vi "main.vi"() -> ()   [LabVIEW 2020]
doc: "该范例演示了通过VI查看其它VI的方法，还可运行和中止查看的VI。\n对于要中止的VI，应设置为可中止。对于无法中止的VI，可查看相关范例。"
uses:
  global/GlobalVariable.vi
  global/SettingVariable.vi
  <vilib>/Utility/config.llb/Write Key (Path).vi
  utilities/NI_modbus.llb/MB Ethernet Master Query Write Multiple Registers (poly).vi
  utilities/NI_modbus.llb/MB Ethernet Master Query Read Input Registers (poly).vi
  <vilib>/Utility/config.llb/NI_LVConfig.lvlib
panel:
  in  "退出":bool
  in  "Measure Square":bool
  in  "Physics Parameters Square":bool
  in  "Open Square":bool
  in  "Home Square":bool
  out "时间":string
  out "日期":string
  in  "MainPanel":enum32{"logo"}(tab)
  out "P2_8":dbl
  out "P2_7":dbl
  out "P2_6":dbl
  out "P2_5":dbl
  out "P2_4":dbl
  out "P2_3":dbl
  out "P2_2":dbl
  out "P2_1":dbl
  out "电流 2":dbl(slide)=1.0 scale=1e-13..0.0001 scale format="%#_2e"
  out "电流 1":dbl(slide)=1.0 scale=1e-13..0.0001 scale format="%#_2e"
  out "电压8":dbl(knob) caption="Gauge" scale=1.0..5.0
  out "电压7":dbl(knob)=1.0 caption="Gauge" scale=1.0..5.0
  out "电压6":dbl(knob)=1.0 caption="Gauge" scale=1.0..5.0
  out "电压5":dbl(knob)=1.0 caption="Gauge" scale=1.0..5.0
  out "电压4":dbl(knob)=1.0 caption="Gauge" scale=1.0..5.0
  out "电压3":dbl(knob)=1.0 caption="Gauge" scale=1.0..5.0
  out "电压2":dbl(knob) caption="Gauge" scale=1.0..5.0
  out "电压1":dbl(knob) caption="Gauge" scale=1.0..5.0
  in  "网络链接":bool
  # "iRho-100型反应性仪"
  # "Network"
  # "Current1"
  # "Current2"
  # "Voltage Output"
  # "Voltage Input"
  # "AC220V/50Hz"
  # "Ground"
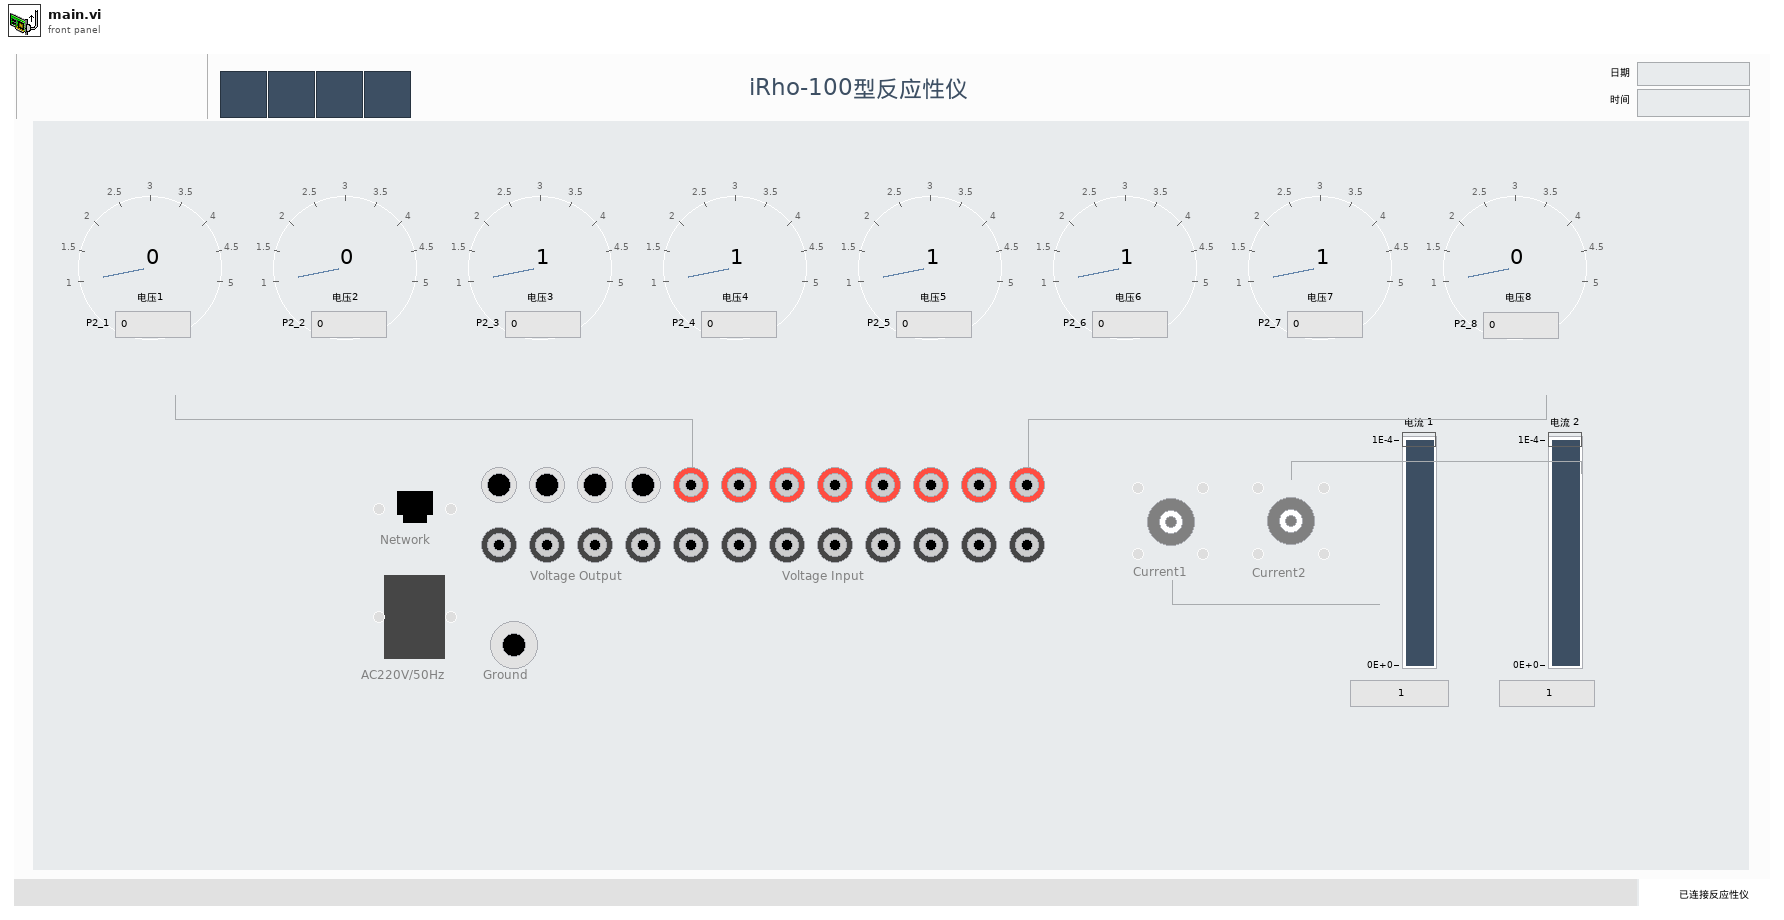
[diagram p1: front panel]
types:
  T1 = enum8{"Enabled", "Disabled", "Disabled and Grayed Out"}
  T2 = enum32{"Invalid", "Standard", "Closed", "Hidden", "Minimized", "Maximized"}
  T3 = cluster{"switch":bool, "name":string, "voltage upper":i32, "voltage lower":i32, "physics upper":dbl, "physics lower":dbl, "scale":u16}[]
  T4 = typedef "NI_LVConfig.lvlib/Config Data RefNum.ctl" = refnum<k1>
  T5 = enum32{"invalid app kind", "Development System", "Run Time System", "Student Edition", "Embedded LabVIEW", "Evaluation", "Custom"}
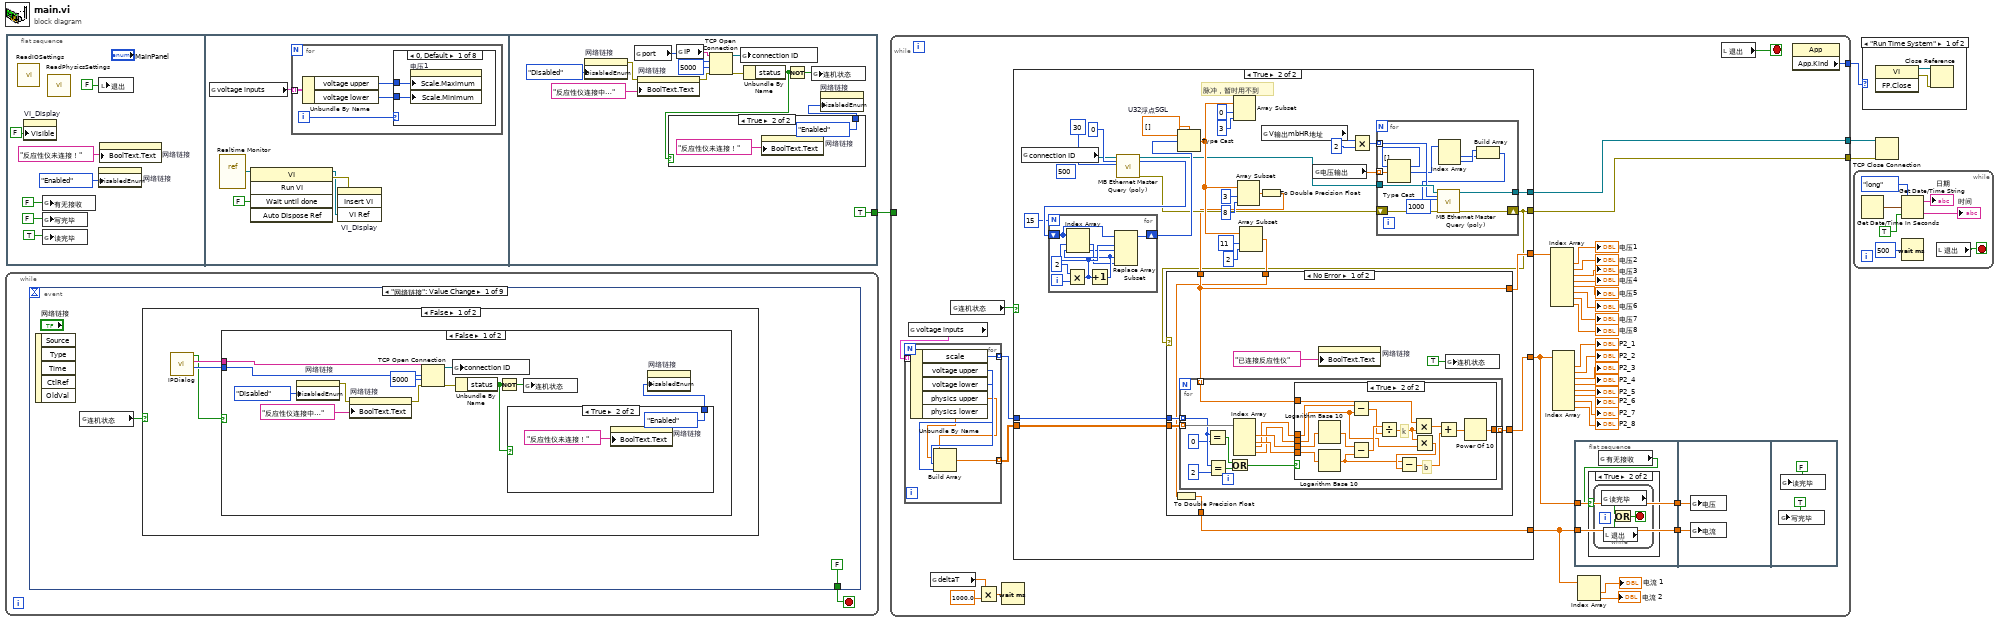
[diagram p0: block diagram]
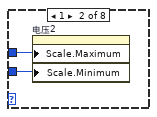
[diagram p2: hidden frame]
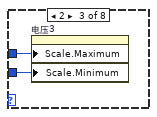
[diagram p3: hidden frame]
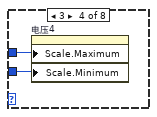
[diagram p4: hidden frame]
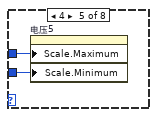
[diagram p5: hidden frame]
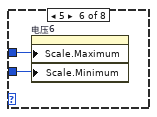
[diagram p6: hidden frame]
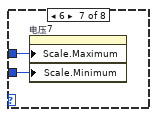
[diagram p7: hidden frame]
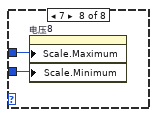
[diagram p8: hidden frame]
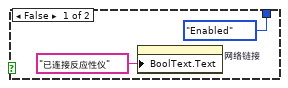
[diagram p9: hidden frame]
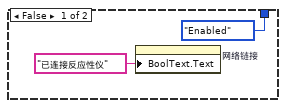
[diagram p10: hidden frame]
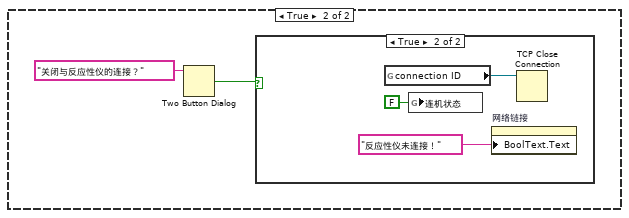
[diagram p12: hidden frame]
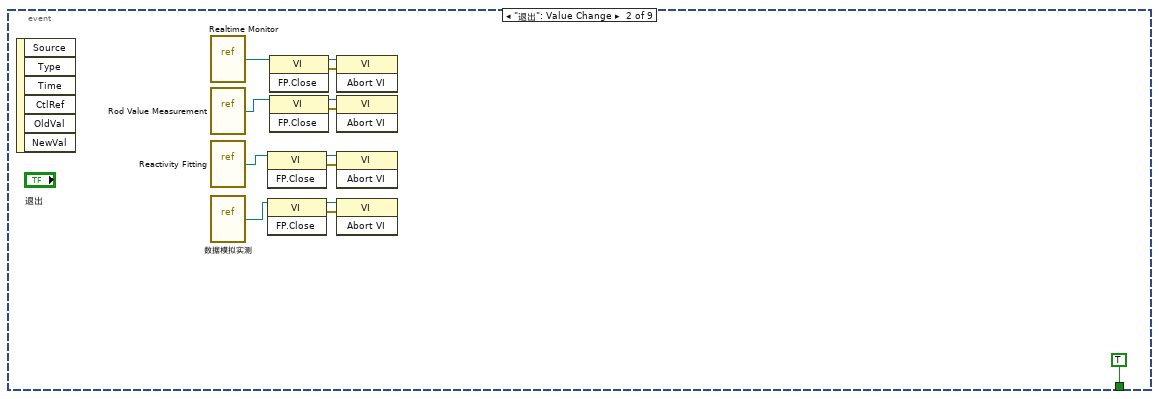
[diagram p14: hidden frame]
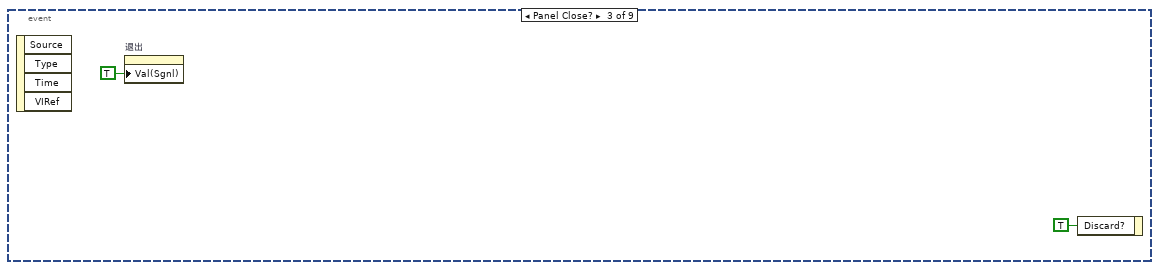
[diagram p15: hidden frame]
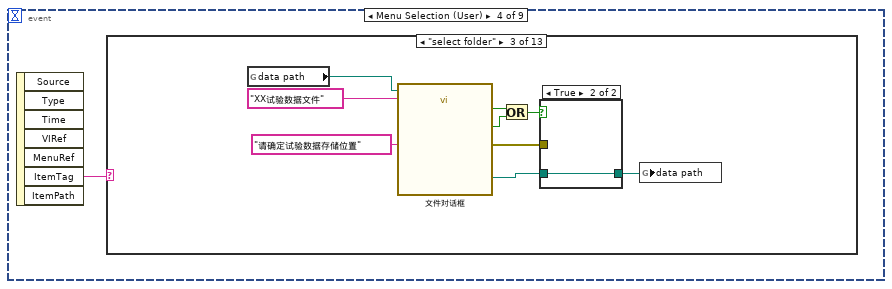
[diagram p16: hidden frame]
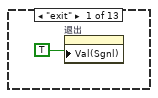
[diagram p17: hidden frame]
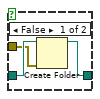
[diagram p19: hidden frame]
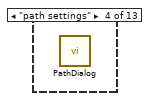
[diagram p20: hidden frame]
diagram:
  n1 = while {
    stop <- w5 stop-if-true
    n2 = event shown="[0] \"网络链接\": Value Change" {
      selector: _ -> [_ _ _ _ _ _ _ _ _]
      dyn-events: _ -> [_ _ _ _ _ _ _ _ _]
      timeout: _ -> [_ _ _ _ _ _ _ _ _]
      tunnel: [FALSE TRUE _ _ _ _ _ _ _] -> w5
      event "网络链接": Value Change {
        n3 = event-data() -> ()  [unwired: 1 in, 5 out]
        n4 = global read "GlobalVariable.vi" "连机状态"() -> (w6:bool)
        n5 = case shown="False" w6 {
          frame False {
            n6 = call "IPDialog.vi"() -> ("port"=w10:u16, "IP"=w9:string, "Cancelled?"=w8:bool)  [unwired: 9 in]
            n7 = case shown="False" w8 {
              tunnel: w10 -> [w14 _]
              tunnel: w9 -> [w13 _]
              frame False {
                n8 = property on="网络链接" class="Bool"("DisabledEnum"=T1."Disabled" ("Disabled")) -> (error out=w17:errorcluster)  [unwired: 2 in, 1 out]
                n9 = property on="网络链接" class="Bool"(error in=w17, "BoolText.Text"="反应性仪连接中…" ("Boolean Text.Text")) -> (error out=w19:errorcluster)  [unwired: 1 in, 1 out]
                n10 = TCP Open Connection(address=w13, remote port or service name=w14, timeout ms (60000)=5000, error in (no error)=w19) -> (connection ID=w18:refnum<k5>, error out=w15:errorcluster)  [unwired: 1 out]
                n11 = global write "GlobalVariable.vi" "connection ID"(w18) -> ()
                n12 = Unbundle By Name(w15) -> ("status"=w20:bool)
                n13 = Not(x=w20) -> (.not. x?=w21:bool)
                n14 = case shown="True" w20 {
                  tunnel: [T1."Enabled" ("Disabled") T1."Enabled" ("Disabled")] -> w12
                  frame False {
                    n15 = property on="网络链接" class="Bool"("BoolText.Text"="已连接反应性仪") -> ()  [unwired: 2 in, 2 out]
                  }
                  frame True {
                    n16 = property on="网络链接" class="Bool"("BoolText.Text"="反应性仪未连接！") -> ()  [unwired: 2 in, 2 out]
                  }
                }
                n17 = global write "GlobalVariable.vi" "连机状态"(w21) -> ()
                n18 = property on="网络链接" class="Bool"("DisabledEnum"=w12) -> ()  [unwired: 2 in, 2 out]
              }
              frame True {
              }
            }
          }
          frame True {
            n19 = Two Button Dialog(message="关闭与反应性仪的连接？") -> (T button?=w27:bool)  [unwired: 2 in]
            n20 = case shown="True" w27 {
              frame False {
              }
              frame True {
                n21 = global read "GlobalVariable.vi" "connection ID"() -> (w31:refnum<k5>)
                n22 = global write "GlobalVariable.vi" "连机状态"(FALSE ("连机状态")) -> ()
                n23 = property on="网络链接" class="Bool"("BoolText.Text"="反应性仪未连接！" ("Boolean Text.Text")) -> ()  [unwired: 2 in, 2 out]
                n24 = TCP Close Connection ("关闭TCP连接")(connection ID=w31) -> ()  [unwired: 1 in, 3 out]
              }
            }
          }
        }
      }
      event "退出": Value Change {
        n25 = event-data() -> ()  [unwired: 1 in, 6 out]
        n26 = vi-ref "Realtime Monitor.vi"() -> (w43:refnum<vi>)
        n27 = vi-ref "Rod Value Measurement.vi"() -> (w42:refnum<vi>)
        n28 = vi-ref "Reactivity Fitting.vi"() -> (w40:refnum<vi>)
        n29 = vi-ref "数据模拟实测.vi"() -> (w41:refnum<vi>)
        n30 = invoke class="VI" method="FP.Close"(reference=w40) -> (reference out=w35:refnum<vi>, error out=w34:errorcluster)  [unwired: 2 in, 1 out]
        n31 = invoke class="VI" method="FP.Close"(reference=w41) -> (reference out=w33:refnum<vi>, error out=w32:errorcluster)  [unwired: 2 in, 1 out]
        n32 = invoke class="VI" method="FP.Close"(reference=w43) -> (reference out=w39:refnum<vi>, error out=w38:errorcluster)  [unwired: 2 in, 1 out]
        n33 = invoke class="VI" method="FP.Close"(reference=w42) -> (reference out=w37:refnum<vi>, error out=w36:errorcluster)  [unwired: 2 in, 1 out]
        n34 = invoke class="VI" method="Abort VI"(reference=w39, error in=w38) -> ()  [unwired: 1 in, 3 out]
        n35 = invoke class="VI" method="Abort VI"(reference=w37, error in=w36) -> ()  [unwired: 1 in, 3 out]
        n36 = invoke class="VI" method="Abort VI"(reference=w35, error in=w34) -> ()  [unwired: 1 in, 3 out]
        n37 = invoke class="VI" method="Abort VI"(reference=w33, error in=w32) -> ()  [unwired: 1 in, 3 out]
      }
      event Panel Close? {
        n38 = event-data() -> ()  [unwired: 1 in, 4 out]
        n39 = property on="退出" class="Bool (strict)"("Val(Sgnl)"=TRUE ("Value (Signaling)")) -> ()  [unwired: 2 in, 2 out]
        n40 = event-data("Discard?"=TRUE) -> ()  [unwired: 1 in, 1 out]
      }
      event Menu Selection (User) {
        n41 = event-data() -> ("ItemTag"=w47:string)  [unwired: 1 in, 6 out]
        n42 = case shown="\"select folder\"" w47 {
          frame "exit" {
            n43 = property on="退出" class="Bool (strict)"("Val(Sgnl)"=TRUE) -> ()  [unwired: 2 in, 2 out]
          }
          frame Default {
          }
          frame "select folder" {
            n44 = global read "SettingVariable.vi" "data path"() -> (w50:path)
            n45 = call "文件对话框"("start path"=w50, "prompt"="请确定试验数据存储位置", "default name"="XX试验数据文件") -> ("selected path"=w57:path, "exists"=w55:bool, "cancelled"=w53:bool, "error out"=w56:errorcluster)  [unwired: 9 in]
            n46 = Or(x=w55, y=w53) -> (x .or. y?=w54:bool)
            n47 = case shown="True" w54 {
              tunnel: w57 -> [w60 w61]
              tunnel: w56 -> [w59 _]
              tunnel: [w58 w61] -> w49
              frame False {
                n48 = Create Folder(path (use dialog)=w60, error in=w59) -> (created path=w58:path)  [unwired: 1 in, 2 out]
              }
              frame True {
              }
            }
            n49 = global write "SettingVariable.vi" "data path"(w49) -> ()
          }
          frame "path settings" {
            n50 = call "PathDialog.vi"() -> ()  [unwired: 11 in, 1 out]
          }
          frame "physics settings" {
            n51 = call "PhysicsDialog.vi"() -> ()  [unwired: 1 in]
          }
          frame "input settings" {
            n52 = call "InputDialog.vi"() -> ("Cancelled?"=w62:bool)  [unwired: 9 in]
            n53 = case shown="True" w62 {
              frame False {
              }
              frame True {
                n54 = global read "SettingVariable.vi" "voltage inputs"() -> (w63:T3)
                n55 = for {
                  tunnel: w63 -> [w67] mode=indexing
                  i -> [w66]
                  n56 = Unbundle By Name(w67) -> ("voltage upper"=w65:i32, "voltage lower"=w64:i32)
                  n57 = case shown="0, Default" w66 {
                    tunnel: w65 -> [w69 w71 w73 w75 w77 w79 w81 w83]
                    tunnel: w64 -> [w68 w70 w72 w74 w76 w78 w80 w82]
                    frame 0, Default {
                      n58 = property on="电压1" class="Knob (strict)"("Scale.Maximum"=w69, "Scale.Minimum"=w68) -> ()  [unwired: 2 in, 2 out]
                    }
                    frame 1 {
                      n59 = property on="电压2" class="Knob (strict)"("Scale.Maximum"=w71, "Scale.Minimum"=w70) -> ()  [unwired: 2 in, 2 out]
                    }
                    frame 2 {
                      n60 = property on="电压3" class="Knob (strict)"("Scale.Maximum"=w73, "Scale.Minimum"=w72) -> ()  [unwired: 2 in, 2 out]
                    }
                    frame 3 {
                      n61 = property on="电压4" class="Knob (strict)"("Scale.Maximum"=w75, "Scale.Minimum"=w74) -> ()  [unwired: 2 in, 2 out]
                    }
                    frame 4 {
                      n62 = property on="电压5" class="Knob (strict)"("Scale.Maximum"=w77, "Scale.Minimum"=w76) -> ()  [unwired: 2 in, 2 out]
                    }
                    frame 5 {
                      n63 = property on="电压6" class="Knob (strict)"("Scale.Maximum"=w79, "Scale.Minimum"=w78) -> ()  [unwired: 2 in, 2 out]
                    }
                    frame 6 {
                      n64 = property on="电压7" class="Knob (strict)"("Scale.Maximum"=w81, "Scale.Minimum"=w80) -> ()  [unwired: 2 in, 2 out]
                    }
                    frame 7 {
                      n65 = property on="电压8" class="Knob (strict)"("Scale.Maximum"=w83, "Scale.Minimum"=w82) -> ()  [unwired: 2 in, 2 out]
                    }
                  }
                }
              }
            }
          }
          frame "output settings" {
            n66 = call "OutputDialog.vi"() -> ()  [unwired: 11 in, 1 out]
          }
          frame "homepage" {
            n67 = property on="VI_Display" class="SubPnl"("Visible"=FALSE) -> ()  [unwired: 2 in, 2 out]
          }
          frame "monitor" {
            n68 = property on="VI_Display" class="SubPnl"("Visible"=TRUE) -> ()  [unwired: 2 in, 2 out]
          }
          frame "rod measurement" {
            n69 = vi-ref "Rod Value Measurement.vi"() -> (w88:refnum<vi>)
            n70 = invoke class="VI" method="FP.Open"(reference=w88, "Activate"=TRUE ("Activate?"), "State"=T2."Standard") -> (reference out=w89:refnum<vi>)  [unwired: 2 in, 4 out]
            n71 = invoke class="VI" method="Run VI"(reference=w89, "Wait until done"=FALSE ("Wait Until Done"), "Auto Dispose Ref"=FALSE ("Auto Dispose Reference")) -> ()  [unwired: 2 in, 5 out]
          }
          frame "reactivity fitting" {
            n72 = vi-ref "Reactivity Fitting.vi"() -> (w94:refnum<vi>)
            n73 = invoke class="VI" method="FP.Open"(reference=w94, "Activate"=TRUE ("Activate?"), "State"=T2."Standard") -> (reference out=w95:refnum<vi>)  [unwired: 2 in, 4 out]
            n74 = invoke class="VI" method="Run VI"(reference=w95, "Wait until done"=FALSE ("Wait Until Done"), "Auto Dispose Ref"=FALSE ("Auto Dispose Reference")) -> ()  [unwired: 2 in, 5 out]
          }
          frame "history simulation" {
            n75 = vi-ref "数据模拟实测.vi"() -> (w100:refnum<vi>)
            n76 = invoke class="VI" method="FP.Open"(reference=w100, "Activate"=TRUE ("Activate?"), "State"=T2."Standard") -> (reference out=w101:refnum<vi>)  [unwired: 2 in, 4 out]
            n77 = invoke class="VI" method="Run VI"(reference=w101, "Wait until done"=FALSE ("Wait Until Done"), "Auto Dispose Ref"=FALSE ("Auto Dispose Reference")) -> ()  [unwired: 2 in, 5 out]
          }
          frame "about" {
            n78 = call "About.vi"() -> ()  [unwired: 1 in]
          }
        }
      }
      event "Home Square": Value Change {
        n79 = event-data() -> ()  [unwired: 1 in, 6 out]
        n80 = property on="VI_Display" class="SubPnl"("Visible"=FALSE) -> ()  [unwired: 2 in, 2 out]
      }
      event "Measure Square": Value Change {
        n81 = event-data() -> ()  [unwired: 1 in, 6 out]
        n82 = property on="VI_Display" class="SubPnl"("Visible"=TRUE) -> ()  [unwired: 2 in, 2 out]
      }
      event "Open Square": Value Change {
        n83 = event-data() -> ()  [unwired: 1 in, 6 out]
        n84 = global read "SettingVariable.vi" "data path"() -> (w106:path)
        n85 = call <vilib>:"Space Constant.vi"() -> ("String"=w120:string)
        n86 = Path To String(path=w106) -> (string=w117:string)
        n87 = Concatenate Strings("explorer" ("字符串"), w120, w117) -> (w118:string)
        n88 = call <vilib>:"System Exec.vi"("command line"=w118) -> ()  [unwired: 7 in, 4 out]
        n89 = call <vilib>:"Application Directory.vi"() -> ("Application Directory"=w112:path)
        n90 = Build Path(base path=w112, name or relative path=path "configure.ini") -> (appended path=w113:path)
        n91 = call <vilib>:"Open Config Data.vi"("configuration file path"=w113) -> ("error out"=w115:errorcluster, "refnum"=w114:T4)  [unwired: 2 in, 7 out]
        n92 = call-poly <vilib>:"Write Key.vi"("section"="Path", "error in (no error)"=w115, "value"=w106, "key"="data" ("section"), "refnum"=w114) -> ("error out"=w110:errorcluster, "refnum out"=w111:T4)  [unwired: 4 in, 1 out]
        n93 = call <vilib>:"Close Config Data.vi"("error in (no error)"=w110, "refnum"=w111) -> ("error out"=w116:errorcluster)  [unwired: 1 in, 8 out]
        n94 = call <vilib>:"Simple Error Handler.vi"("error in (no error)"=w116) -> ()  [unwired: 1 in, 8 out]
      }
      event "Physics Parameters Square": Value Change {
        n95 = event-data() -> ()  [unwired: 1 in, 6 out]
        n96 = call "PhysicsDialog.vi"() -> ()  [unwired: 1 in]
      }
      event "时间": Shortcut Menu Selection (User) {
        n97 = event-data() -> ("ItemTag"=w121:string)  [unwired: 1 in, 7 out]
        n98 = case shown="\"time calibration\", Default" w121 {
          frame "time calibration", Default {
            n99 = global read "GlobalVariable.vi" "连机状态"() -> (w122:bool)
            n100 = case shown="True" w122 {
              frame False {
                n101 = One Button Dialog(message="未连接反应性仪") -> ()  [unwired: 1 in, 1 out]
              }
              frame True {
                w130 = "%x" ("格式字符串")
                w131 = u16[] [] ("数组类型(2D Dbl)")
                n102 = Get Date/Time String(want seconds? (F)=TRUE ("需要秒？(F)")) -> (date string=w147:string, time string=w146:string)  [unwired: 2 in]
                n103 = Spreadsheet String To Array(delimiter (Tab)="/" ("分隔符(Tab)"), format string=w130, spreadsheet string=w147, array type (2D Dbl)=w131) -> (array=w143:u16[])
                n104 = Spreadsheet String To Array(delimiter (Tab)=":" ("分隔符(Tab)"), format string=w130, spreadsheet string=w146, array type (2D Dbl)=w131) -> (array=w141:u16[])
                n105 = Index Array(array=w143, index=0 ("索引")) -> (element=w145:u16)
                n106 = Subtract(x=w145, y=u16 8192) -> (x-y=w144:u16)
                n107 = Replace Array Subset(array=w143, new element=w144, index=0 ("索引")) -> (w142:u16[])
                n108 = Build Array (concatenate)(w142, w141) -> (w140:u16[])
                n109 = To Unsigned Byte Integer(number=w140) -> (unsigned 8bit integer=w139:u8[])
                n110 = for {
                  N: 3 -> [_]
                  shift-right: [w149] -> w138
                  shift-left: w139 -> [w154]
                  i -> [w156]
                  n111 = Multiply(x=2, y=w156) -> (x*y=w153:i32)
                  n112 = Increment(x=w153) -> (x+1=w152:i32)
                  n113 = Index Array(array=w154, index #1=w153, index #2=w152) -> (element #1=w151:u8, element #2=w150:u8)
                  n114 = Replace Array Subset(array=w154, new element #1=w150, index #1=w153, new element #2=w151, index #2=w152) -> (w149:u8[])
                }
                n115 = global read "GlobalVariable.vi" "connection ID"() -> (w124:refnum<k5>)
                n116 = Type Cast(type=u16[] [] ("Input Registers"), x=w138) -> (*(type *) &x=w126:u16[])
                n117 = call-poly "MB Ethernet Master Query (poly).vi"("TCP Connection Refnum in"=w124, "Starting Address"=u16 65436, "Registers"=w126) -> ("error out"=w125:errorcluster)  [unwired: 3 in, 13 out]
                n118 = case shown="Error .." w125 {
                  frame No Error {
                  }
                  frame Error {
                    n119 = One Button Dialog(message="写入失败！请检查网络连接。") -> ()  [unwired: 1 in, 1 out]
                  }
                }
              }
            }
          }
        }
      }
    }
  }
  n120 = flat-sequence {
    tunnel: [TRUE] -> w1
    frame #0 {
      n121 = call "ReadIOSettings.vi"() -> ()  [unwired: 12 in]
      n122 = property on="VI_Display" class="SubPnl"("Visible"=FALSE) -> ()  [unwired: 2 in, 2 out]
      n123 = global write "GlobalVariable.vi" "有无接收"(FALSE ("读完毕")) -> ()
      n124 = global write "GlobalVariable.vi" "写完毕"(FALSE ("读完毕")) -> ()
      n125 = global write "GlobalVariable.vi" "读完毕"(TRUE ("读完毕")) -> ()
      n126 = call "ReadPhysicsSettings.vi"() -> ()  [unwired: 12 in]
      n127 = local write "退出"(FALSE ("退出")) -> ()
      n128 = property on="网络链接" class="Bool"("DisabledEnum"=T1."Enabled" ("Disabled")) -> ()  [unwired: 2 in, 2 out]
      n129 = property on="网络链接" class="Bool"("BoolText.Text"="反应性仪未连接！") -> ()  [unwired: 2 in, 2 out]
    }
    frame #1 {
      n130 = global read "SettingVariable.vi" "voltage inputs"() -> (w168:T3)
      n131 = vi-ref "Realtime Monitor.vi"() -> (w165:refnum<vi>)
      n132 = invoke class="VI" method="Run VI"(reference=w165, "Wait until done"=FALSE ("Wait Until Done")) -> (reference out=w166:refnum<vi>, error out=w167:errorcluster)  [unwired: 3 in, 3 out]
      n133 = for {
        tunnel: w168 -> [w172] mode=indexing
        i -> [w171]
        n134 = Unbundle By Name(w172) -> ("voltage upper"=w170:i32, "voltage lower"=w169:i32)
        n135 = case shown="0, Default" w171 {
          tunnel: w170 -> [w174 w176 w178 w180 w182 w184 w186 w188]
          tunnel: w169 -> [w173 w175 w177 w179 w181 w183 w185 w187]
          frame 0, Default {
            n136 = property on="电压1" class="Knob (strict)"("Scale.Maximum"=w174, "Scale.Minimum"=w173) -> ()  [unwired: 2 in, 2 out]
          }
          frame 1 {
            n137 = property on="电压2" class="Knob (strict)"("Scale.Maximum"=w176, "Scale.Minimum"=w175) -> ()  [unwired: 2 in, 2 out]
          }
          frame 2 {
            n138 = property on="电压3" class="Knob (strict)"("Scale.Maximum"=w178, "Scale.Minimum"=w177) -> ()  [unwired: 2 in, 2 out]
          }
          frame 3 {
            n139 = property on="电压4" class="Knob (strict)"("Scale.Maximum"=w180, "Scale.Minimum"=w179) -> ()  [unwired: 2 in, 2 out]
          }
          frame 4 {
            n140 = property on="电压5" class="Knob (strict)"("Scale.Maximum"=w182, "Scale.Minimum"=w181) -> ()  [unwired: 2 in, 2 out]
          }
          frame 5 {
            n141 = property on="电压6" class="Knob (strict)"("Scale.Maximum"=w184, "Scale.Minimum"=w183) -> ()  [unwired: 2 in, 2 out]
          }
          frame 6 {
            n142 = property on="电压7" class="Knob (strict)"("Scale.Maximum"=w186, "Scale.Minimum"=w185) -> ()  [unwired: 2 in, 2 out]
          }
          frame 7 {
            n143 = property on="电压8" class="Knob (strict)"("Scale.Maximum"=w188, "Scale.Minimum"=w187) -> ()  [unwired: 2 in, 2 out]
          }
        }
      }
      n144 = invoke on="VI_Display" class="SubPnl" method="Insert VI"(error in=w167, "VI Ref"=w166) -> ()  [unwired: 2 in, 4 out]
    }
    frame #2 {
      n145 = property on="网络链接" class="Bool"("DisabledEnum"=T1."Disabled" ("Disabled")) -> (error out=w199:errorcluster)  [unwired: 2 in, 1 out]
      n146 = global read "SettingVariable.vi" "port"() -> (w191:u16)
      n147 = property on="网络链接" class="Bool"(error in=w199, "BoolText.Text"="反应性仪连接中…" ("Boolean Text.Text")) -> (error out=w197:errorcluster)  [unwired: 1 in, 1 out]
      n148 = global read "SettingVariable.vi" "IP"() -> (w192:string)
      n149 = TCP Open Connection(address=w192, remote port or service name=w191, timeout ms (60000)=5000, error in (no error)=w197) -> (connection ID=w198:refnum<k5>, error out=w201:errorcluster)  [unwired: 1 out]
      n150 = global write "GlobalVariable.vi" "connection ID"(w198) -> ()
      n151 = Unbundle By Name(w201) -> ("status"=w194:bool)
      n152 = case shown="True" w194 {
        tunnel: [T1."Enabled" ("Disabled") T1."Enabled" ("Disabled")] -> w193
        frame False {
          n153 = property on="网络链接" class="Bool"("BoolText.Text"="已连接反应性仪") -> ()  [unwired: 2 in, 2 out]
        }
        frame True {
          n154 = property on="网络链接" class="Bool"("BoolText.Text"="反应性仪未连接！") -> ()  [unwired: 2 in, 2 out]
        }
      }
      n155 = Not(x=w194) -> (.not. x?=w195:bool)
      n156 = global write "GlobalVariable.vi" "连机状态"(w195) -> ()
      n157 = property on="网络链接" class="Bool"("DisabledEnum"=w193) -> ()  [unwired: 2 in, 2 out]
    }
  }
  n158 = while {
    tunnel: [w212] -> w3
    tunnel: [w211] -> w2
    tunnel: [w214] -> w4
    tunnel: w1 -> [_]
    stop <- w213 stop-if-true
    n159 = global read "SettingVariable.vi" "voltage inputs"() -> (w209:T3)
    n160 = for {
      tunnel: w209 -> [w246] mode=indexing
      tunnel: [w245] -> w208 mode=indexing
      tunnel: [w240] -> w207 mode=indexing
      n161 = Unbundle By Name(w246) -> ("scale"=w245:u16, "voltage upper"=w244:i32, "voltage lower"=w243:i32, "physics upper"=w242:dbl, "physics lower"=w241:dbl)
      n162 = Build Array(w242, w241, w244, w243) -> (w240:dbl[])
    }
    n163 = global read "SettingVariable.vi" "deltaT"() -> (w210:dbl)
    n164 = global read "GlobalVariable.vi" "连机状态"() -> (w206:bool)
    n165 = Multiply(x=w210, y=1000.0) -> (x*y=w216:dbl)
    n166 = Wait (ms)(milliseconds to wait=w216) -> ()  [unwired: 1 out]
    n167 = case shown="True" w206 {
      tunnel: w208 -> [_ w260]
      tunnel: w207 -> [_ w261]
      tunnel: [dbl[] [nan, nan, nan, nan, nan, nan, nan, nan] w259] -> w237
      tunnel: [dbl[] [nan, nan] w256] -> w236
      tunnel: [dbl[] [nan, nan, nan, nan, nan, nan, nan, nan] w262] -> w215
      tunnel: [w251 w264] -> w212
      tunnel: [errorcluster {"status"=FALSE, "code"=0, "source"=""} ("error out") w252] -> w211
      frame False {
        n168 = global read "GlobalVariable.vi" "connection ID"() -> (w251:refnum<k5>)
      }
      frame True {
        (unwired) 500 ("Timeout")
        w271 = sgl[] []  # U32浮点SGL
        # "脉冲，暂时用不到"
        n169 = global read "GlobalVariable.vi" "connection ID"() -> (w266:refnum<k5>)
        n170 = call-poly "MB Ethernet Master Query (poly).vi"("TCP Connection Refnum in"=w266, "Starting Address"=u16 0, "Quantity"=u16 30 ("modbus寄存器数量")) -> ("TCP Connection Refnum (dup)"=w265:refnum<k5>, "Input Registers"=w269:u16[], "error out"=w263:errorcluster)  [unwired: 2 in, 12 out]
        n171 = for {
          N: 15 -> [_]
          shift-right: [w282] -> w268
          shift-left: w269 -> [w287]
          i -> [w289]
          n172 = Multiply(x=2, y=w289) -> (x*y=w286:i32)
          n173 = Increment(x=w286) -> (x+1=w285:i32)
          n174 = Index Array(array=w287, index #1=w286, index #2=w285) -> (element #1=w284:u16, element #2=w283:u16)
          n175 = Replace Array Subset(array=w287, new element #1=w283, index #1=w286, new element #2=w284, index #2=w285) -> (w282:u16[])
        }
        n176 = Type Cast(type=w271, x=w268) -> (*(type *) &x=w274:sgl[])
        n177 = Array Subset(array=w274, index=0 ("索引"), length=3 ("长度")) -> ()  [unwired: 1 out]
        n178 = Array Subset(array=w274, index=3 ("索引"), length=8 ("长度")) -> (w277:sgl[])
        n179 = Array Subset(array=w274, index=11 ("索引"), length=2 ("长度")) -> (w257:sgl[])
        n180 = To Double Precision Float(number=w277) -> (double precision float=w258:dbl[])
        n181 = global read "GlobalVariable.vi" "V输出mbHR地址"() -> (w254:u16[])
        n182 = global read "GlobalVariable.vi" "电压输出"() -> (w273:sgl[])
        n183 = Multiply(x=w254, y=2) -> (x*y=w255:i32[])
        n184 = for {
          tunnel: w265 -> [w299]
          tunnel: [w297] -> w264
          tunnel: w273 -> [w296] mode=indexing
          tunnel: w255 -> [w295] mode=indexing
          shift-right: [w298] -> w252
          shift-left: w263 -> [w300]
          (unwired) u32 1000 ("Timeout")
          n185 = Type Cast(type=u16[] [] ("Input Registers"), x=w296) -> (*(type *) &x=w293:u16[])
          n186 = Index Array(array=w293) -> (element #1=w290:u16, element #2=w291:u16)  [unwired: 2 in]
          n187 = Build Array(w291, w290) -> (w292:u16[])
          n188 = call-poly "MB Ethernet Master Query (poly).vi"("TCP Connection Refnum in"=w299, "Starting Address"=w295, "Registers"=w292, "error in"=w300) -> ("TCP Connection Refnum (dup)"=w297:refnum<k5>, "error out"=w298:errorcluster)  [unwired: 2 in, 12 out]
        }
        n189 = case shown="No Error" w252 {
          tunnel: [w308 dbl[] [nan, nan, nan, nan, nan, nan, nan, nan]] -> w262
          tunnel: w258 -> [w308 _]
          tunnel: w261 -> [w307 _]
          tunnel: w260 -> [w306 _]
          tunnel: [w305 dbl[] [nan, nan, nan, nan, nan, nan, nan, nan]] -> w259
          tunnel: w257 -> [w302 _]
          tunnel: [w301 dbl[] [nan, nan]] -> w256
          frame No Error {
            n190 = To Double Precision Float(number=w302) -> (double precision float=w301:dbl[])
            n191 = for {
              tunnel: w308 -> [w320] mode=indexing
              tunnel: [w319] -> w305 mode=indexing
              tunnel: w307 -> [w321] mode=indexing
              tunnel: w306 -> [w318] mode=indexing
              n192 = Equal?(x=w318, y=u16 0) -> (x = y?=w315:bool)
              n193 = Equal?(x=w318, y=u16 2) -> (x = y?=w314:bool)
              n194 = Or(x=w315, y=w314) -> (x .or. y?=w313:bool)
              n195 = Index Array(array=w321) -> (element #1=w312:dbl, element #2=w311:dbl, element #3=w310:dbl, element #4=w309:dbl)  [unwired: 4 in]
              n196 = case shown="True" w313 {
                tunnel: w320 -> [w333 w339]
                tunnel: [w332 w337] -> w319
                tunnel: w310 -> [w325 w342]
                tunnel: w309 -> [w324 w341]
                tunnel: w312 -> [w323 w335]
                tunnel: w311 -> [w322 w340]
                frame False {
                  # "b"
                  # "k"
                  n197 = Subtract(x=w325, y=w324) -> (x-y=w330:dbl)
                  n198 = Subtract(x=w323, y=w322) -> (x-y=w331:dbl)
                  n199 = Divide(x=w331, y=w330) -> (x/y=w329:dbl)
                  n200 = Multiply(x=w333, y=w329) -> (x*y=w327:dbl)
                  n201 = Multiply(x=w329, y=w324) -> (x*y=w328:dbl)
                  n202 = Subtract(x=w322, y=w328) -> (x-y=w326:dbl)
                  n203 = Add(x=w327, y=w326) -> (x+y=w332:dbl)
                }
                frame True {
                  # "b"
                  # "k"
                  n204 = Logarithm Base 10(1:w335) -> (0:w334:dbl)
                  n205 = Logarithm Base 10(1:w340) -> (0:w336:dbl)
                  n206 = Subtract(x=w342, y=w341) -> (x-y=w347:dbl)
                  n207 = Subtract(x=w334, y=w336) -> (x-y=w348:dbl)
                  n208 = Divide(x=w348, y=w347) -> (x/y=w346:dbl)
                  n209 = Multiply(x=w339, y=w346) -> (x*y=w344:dbl)
                  n210 = Multiply(x=w346, y=w341) -> (x*y=w345:dbl)
                  n211 = Subtract(x=w336, y=w345) -> (x-y=w343:dbl)
                  n212 = Add(x=w344, y=w343) -> (x+y=w338:dbl)
                  n213 = Power Of 10(x=w338) -> (10^x=w337:dbl)
                }
              }
            }
            n214 = property on="网络链接" class="Bool"("BoolText.Text"="已连接反应性仪") -> ()  [unwired: 2 in, 2 out]
            n215 = global write "GlobalVariable.vi" "连机状态"(TRUE ("连机状态")) -> ()
          }
          frame Error {
            n216 = property on="网络链接" class="Bool"("BoolText.Text"="反应性仪未连接！") -> ()  [unwired: 2 in, 2 out]
            n217 = global write "GlobalVariable.vi" "连机状态"(FALSE ("连机状态")) -> ()
          }
        }
      }
    }
    n218 = Index Array(array=w215) -> (element #1=→"电压1":dbl, element #2=→"电压2":dbl, element #3=→"电压3":dbl, element #4=→"电压4":dbl, element #5=→"电压5":dbl, element #6=→"电压6":dbl, element #7=→"电压7":dbl, element #8=→"电压8":dbl)  [unwired: 8 in]
    n219 = Index Array(array=w237) -> (element #1=→"P2_1":dbl, element #2=→"P2_2":dbl, element #3=→"P2_3":dbl, element #4=→"P2_4":dbl, element #5=→"P2_5":dbl, element #6=→"P2_6":dbl, element #7=→"P2_7":dbl, element #8=→"P2_8":dbl)  [unwired: 8 in]
    n220 = flat-sequence {
      tunnel: w236 -> [w355]
      tunnel: w237 -> [w356]
      tunnel: [w356] -> w239
      tunnel: [w355] -> w238
      tunnel: w239 -> [w361]
      tunnel: w238 -> [w360]
      frame #0 {
        n221 = global read "GlobalVariable.vi" "有无接收"() -> (w354:bool)
        n222 = case shown="True" w354 {
          frame False {
          }
          frame True {
            n223 = while {
              stop <- w358 stop-if-true
              n224 = global read "GlobalVariable.vi" "读完毕"() -> (w357:bool)
              n225 = local read "退出"() -> (w359:bool)
              n226 = Or(x=w357, y=w359) -> (x .or. y?=w358:bool)
            }
          }
        }
      }
      frame #1 {
        n227 = global write "GlobalVariable.vi" "电压"(w361) -> ()
        n228 = global write "GlobalVariable.vi" "电流"(w360) -> ()
      }
      frame #2 {
        n229 = global write "GlobalVariable.vi" "写完毕"(TRUE ("写完毕")) -> ()
        n230 = global write "GlobalVariable.vi" "读完毕"(FALSE ("写完毕")) -> ()
      }
    }
    n231 = Index Array(array=w236) -> (element #1=→"电流 1":dbl, element #2=→"电流 2":dbl)  [unwired: 2 in]
    n232 = local read "退出"() -> (w213:bool)
    n233 = property class="App"() -> ("App.Kind"=w214:T5)  [unwired: 2 in, 2 out]
  }
  n234 = while {
    stop <- w366 stop-if-true
    n235 = Get Date/Time In Seconds() -> (seconds since 1Jan1904=w370:timestamp)
    n236 = Get Date/Time String(date format (0)=enum16{"short", "long", "abbreviated"}."long" ("日期格式(0)"), seconds (now)=w370, want seconds? (F)=TRUE) -> (date string=→"日期":string, time string=→"时间":string)
    n237 = Wait (ms)(milliseconds to wait=u32 500) -> ()  [unwired: 1 out]
    n238 = local read "退出"() -> (w366:bool)
  }
  n239 = case shown="\"Run Time System\"" w4 {
    frame "Run Time System" {
      n240 = invoke class="VI" method="FP.Close"() -> (reference out=w371:refnum<vi>, error out=w372:errorcluster)  [unwired: 3 in, 1 out]
      n241 = Close Reference(reference=w371, error in (no error)=w372) -> ()  [unwired: 1 out]
    }
    frame "Development System", Default {
    }
  }
  n242 = TCP Close Connection ("关闭TCP连接")(connection ID=w3, error in (no error)=w2) -> ()  [unwired: 3 out]
